vi "Get Visible Frame Config.vi"(7 "pDepth":i32, 9 "pHeight":i32, 10 "pWidth":i32, 11 "index":u16) -> (1 "pHeight out":i32, 2 "pWidth out":i32, 3 "function return":i32, 5 "pDepth out":i32)   [LabVIEW 2025, in "ExtremelyEpicImagerIPC2.lvlib"]
doc: "IMAGERIPC_API HRESULT WINAPI GetVisibleFrameConfig(WORD index, int *pWidth, int *pHeight, int *pDepth);"
uses:
  ExtremelyEpicImagerIPC2.lvlib
  ImagerIPC2.dll
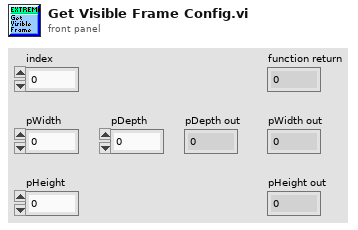
[diagram p1: front panel]
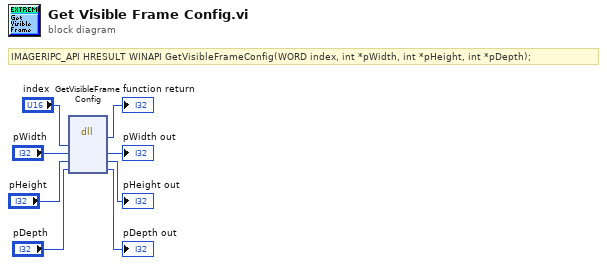
[diagram p0: block diagram]
diagram:
  # "IMAGERIPC_API HRESULT WINAPI GetVisibleFrameConfig(WORD index, int *pWidth, int *pHeight, int *pDepth);"
  n1 = dll-call lib="C:/Users/mayhe/OneDrive/Documents/GitHub/In-situ-monitoring-of-powder-bed-fusion-additive-manufacturing/system_development/Orichalcum/v0.2/Software_design/thermal-camera/VI/Connect SDK/ImagerIPC2.*" fn="GetVisibleFrameConfig"("index"="index", "pWidth"="pWidth", "pHeight"="pHeight", "pDepth"="pDepth") -> (→"function return":i32, "pWidth"=→"pWidth out":i32, "pHeight"=→"pHeight out":i32, "pDepth"=→"pDepth out":i32)  [unwired: 4 in, 2 out]
